vi "Main.vi"(8 "error in":errorcluster, 11 "gRPC Client Tester in":refnum<class "gRPC Client Tester.lvclass">) -> (0 "error out":errorcluster, 3 "gRPC Client Tester out":refnum<class "gRPC Client Tester.lvclass">)   [LabVIEW 2019, in "gRPC Client Tester.lvclass"]
doc: "The <b>Queued Message Handler</b> of the Worker that owns this VI."
uses:
  gRPC Client Tester.lvclass
  C:/Program Files (x86)/National Instruments/LabVIEW 2019/vi.lib/addons/_Workers/Library/Classes/Worker/Worker.lvclass
  Generated_client/RPC Messages/w4lvgrpc_Msg_ToServer_4.ctl
  Generated_client/RPC Messages/w4lvgrpc_Msg_ToServer_1.ctl
  Generated_client/RPC Messages/w4lvgrpc_Msg_ToServer_2.ctl
  Generated_client/RPC Messages/w4lvgrpc_Msg_ToServer_3.ctl
  Generated_client/RPC Messages/w4lvgrpc_Msg_ToServer_5.ctl
  Generated_client/RPC Messages/w4lvgrpc_Msg_ToClient_1.ctl
  Generated_client/RPC Messages/w4lvgrpc_Msg_ToClient_2.ctl
  Generated_client/RPC Messages/w4lvgrpc_Msg_ToClient_3.ctl
  Generated_client/RPC Messages/w4lvgrpc_Msg_ToClient_4.ctl
  Generated_client/RPC Messages/w4lvgrpc_Msg_ToClient_5.ctl
  gRPC Client Tester.lvclass/gRPC Client Tester.ctl
  gRPC Client/gRPC Client/rqp_Msg_ToServer_1.ctl
  gRPC Client/gRPC Client/rqp_Msg_ToServer_2.ctl
  gRPC Client/gRPC Client/rqp_Msg_ToServer_3.ctl
  gRPC Client/gRPC Client/rqp_Msg_ToServer_4.ctl
  gRPC Client/gRPC Client/rqp_Msg_ToServer_5.ctl
  Initialization Data.ctl
  Response Cases.ctl
  rql_Create gRPC Client.ctl
  gRPC Client/gRPC Client/rwr_Create gRPC Client.ctl
  rql_Destroy gRPC Client.ctl
  <vilib>/addons/_Workers/Library/Classes/Message Queue/Message Queue.lvclass
  gRPC Client/gRPC Client/gRPC Client.lvclass
  Generated_client/Generated_client.lvlib
panel:
  out "Msg_ToClient_5":T1
  out "Msg_ToClient_4":T2
  out "Msg_ToClient_3":T3
  out "Msg_ToClient_2":T4
  out "Msg_ToClient_1":T5
  in  "Msg_ToServer_5":T6
  in  "Msg_ToServer_3":T7
  in  "Msg_ToServer_2":T8
  in  "Msg_ToServer_1":T9
  in  "Msg_ToServer_4":T10
  out "gRPC ID":u64
  out "Client Connected":bool
  in  "Server Address":string="localhost:50070"
  in  "Destroy gRPC Client":bool
  in  "Create gRPC Client":bool
  # "gRPC Client Worker - Public Requests"
  # "Messages Client -> Server"
  # "gRPC Client Worker Template Tester"
  # "Instructions:\n\nSee project file called Readme.md"
  # "gRPC Client Worker - Public Responses"
  # "Messages Server -> Client"
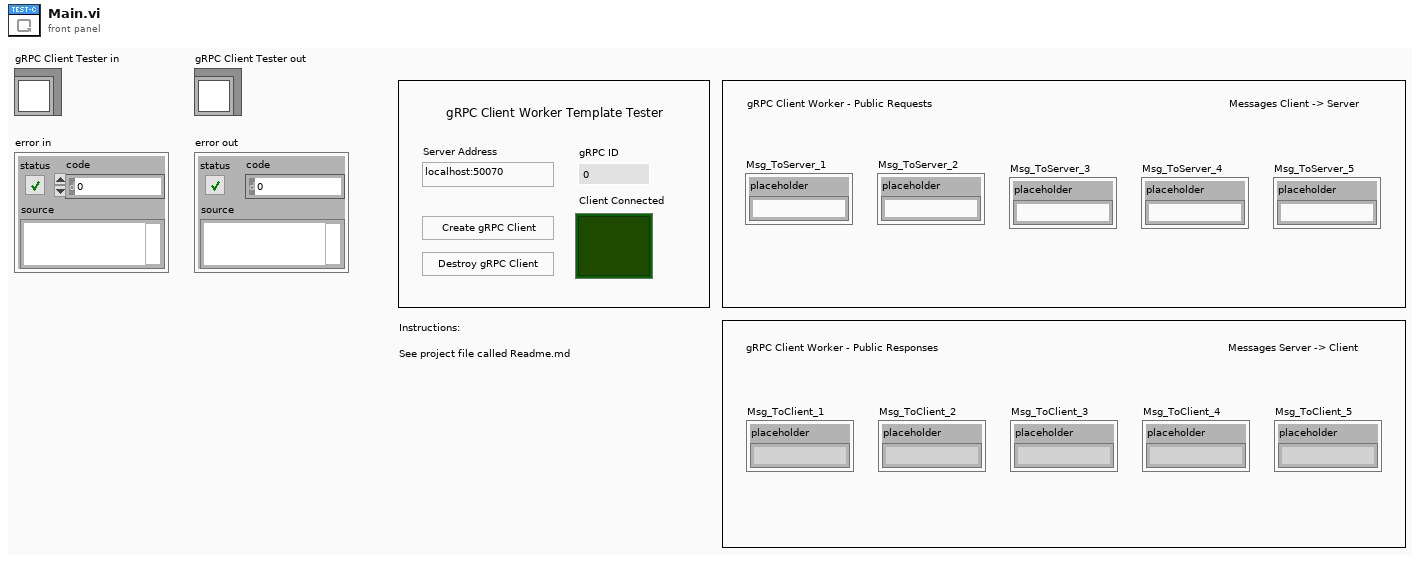
[diagram p1: front panel]
types:
  T1 = typedef "Generated_client.lvlib/w4lvgrpc_Msg_ToClient_5.ctl" = cluster{"placeholder":string}
  T2 = typedef "Generated_client.lvlib/w4lvgrpc_Msg_ToClient_4.ctl" = cluster{"placeholder":string}
  T3 = typedef "Generated_client.lvlib/w4lvgrpc_Msg_ToClient_3.ctl" = cluster{"placeholder":string}
  T4 = typedef "Generated_client.lvlib/w4lvgrpc_Msg_ToClient_2.ctl" = cluster{"placeholder":string}
  T5 = typedef "Generated_client.lvlib/w4lvgrpc_Msg_ToClient_1.ctl" = cluster{"placeholder":string}
  T6 = typedef "Generated_client.lvlib/w4lvgrpc_Msg_ToServer_5.ctl" = cluster{"placeholder":string}
  T7 = typedef "Generated_client.lvlib/w4lvgrpc_Msg_ToServer_3.ctl" = cluster{"placeholder":string}
  T8 = typedef "Generated_client.lvlib/w4lvgrpc_Msg_ToServer_2.ctl" = cluster{"placeholder":string}
  T9 = typedef "Generated_client.lvlib/w4lvgrpc_Msg_ToServer_1.ctl" = cluster{"placeholder":string}
  T10 = typedef "Generated_client.lvlib/w4lvgrpc_Msg_ToServer_4.ctl" = cluster{"placeholder":string}
  T11 = typedef "gRPC Client Tester.lvclass/Initialization Data.ctl" = cluster{"Response Cases":T12}
  T12 = typedef "gRPC Client Tester.lvclass/Response Cases.ctl" = cluster{"Placeholder - Can be deleted":string}
  T13 = typedef "gRPC Client Tester.lvclass/rql_Create gRPC Client.ctl" = cluster{"String":string}
  T14 = typedef "gRPC Client (template.proto).lvlib/gRPC Client.lvclass/rwr_Create gRPC Client.ctl" = cluster{"Server Address":string, "Certificate Path":string}
  T15 = typedef "gRPC Client Tester.lvclass/rql_Destroy gRPC Client.ctl" = cluster{"String":string}
  T16 = typedef "gRPC Client (template.proto).lvlib/gRPC Client.lvclass/rqp_Msg_ToServer_1.ctl" = cluster{"w4lvgrpc_Msg_ToServer_1":T9}
  T17 = typedef "gRPC Client (template.proto).lvlib/gRPC Client.lvclass/rqp_Msg_ToServer_2.ctl" = cluster{"w4lvgrpc_Msg_ToServer_2":T8}
  T18 = typedef "gRPC Client (template.proto).lvlib/gRPC Client.lvclass/rqp_Msg_ToServer_3.ctl" = cluster{"w4lvgrpc_Msg_ToServer_3":T7}
  T19 = typedef "gRPC Client (template.proto).lvlib/gRPC Client.lvclass/rqp_Msg_ToServer_4.ctl" = cluster{"w4lvgrpc_Msg_ToServer_4":T10}
  T20 = typedef "gRPC Client (template.proto).lvlib/gRPC Client.lvclass/rqp_Msg_ToServer_5.ctl" = cluster{"w4lvgrpc_Msg_ToServer_5":T6}
  T21 = typedef "gRPC Client (template.proto).lvlib/gRPC Client.lvclass/rsp_Connection Notify.ctl" = cluster{"gRPC ID":T22, "Connected?":bool}
  T22 = typedef "grpc-lvsupport-release.lvlib/grpcId.ctl" = u64
  T23 = typedef "gRPC Client (template.proto).lvlib/gRPC Client.lvclass/rsp_Client Error.ctl" = errorcluster
  T24 = typedef "gRPC Client (template.proto).lvlib/gRPC Client.lvclass/rsp_Msg_ToClient_1.ctl" = cluster{"w4lvgrpc_Msg_ToClient_1":T5}
  T25 = typedef "gRPC Client (template.proto).lvlib/gRPC Client.lvclass/rsp_Msg_ToClient_2.ctl" = cluster{"w4lvgrpc_Msg_ToClient_2":T4}
  T26 = typedef "gRPC Client (template.proto).lvlib/gRPC Client.lvclass/rsp_Msg_ToClient_3.ctl" = cluster{"w4lvgrpc_Msg_ToClient_3":T3}
  T27 = typedef "gRPC Client (template.proto).lvlib/gRPC Client.lvclass/rsp_Msg_ToClient_4.ctl" = cluster{"w4lvgrpc_Msg_ToClient_4":T2}
  T28 = typedef "gRPC Client (template.proto).lvlib/gRPC Client.lvclass/rsp_Msg_ToClient_5.ctl" = cluster{"w4lvgrpc_Msg_ToClient_5":T1}
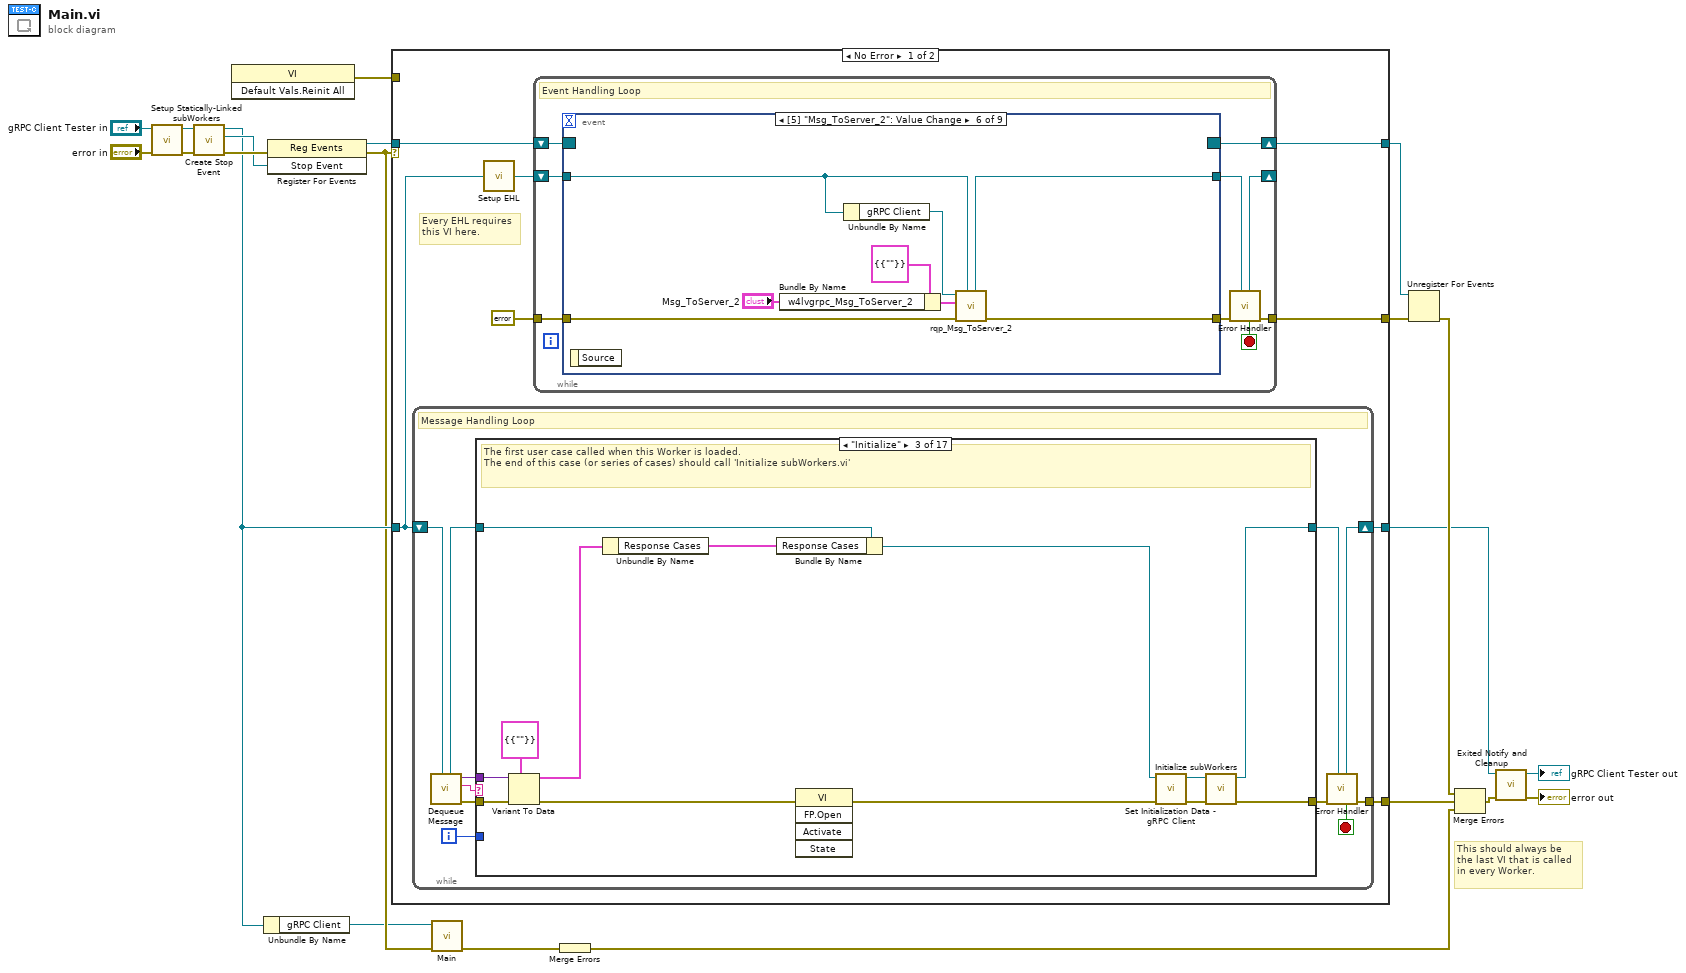
[diagram p0: block diagram]
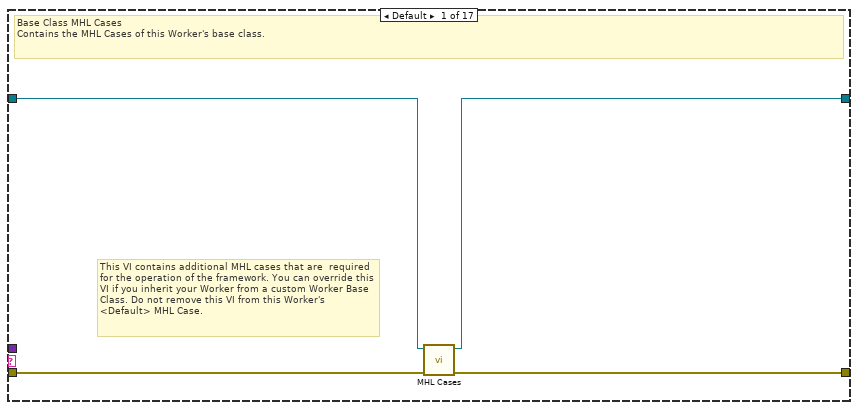
[diagram p2: hidden frame]
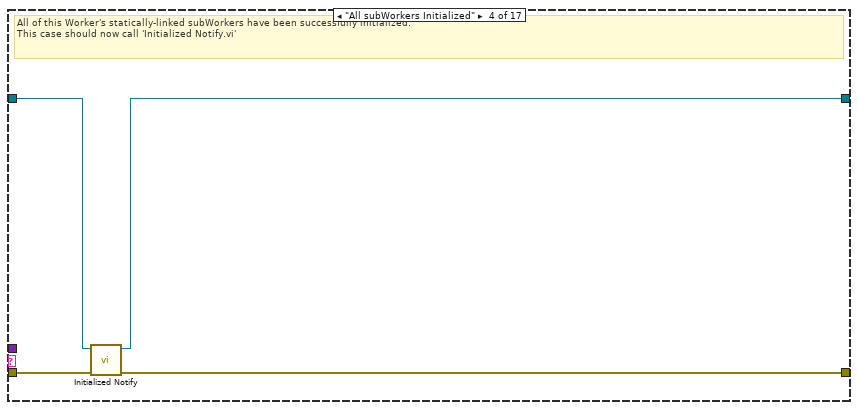
[diagram p4: hidden frame]
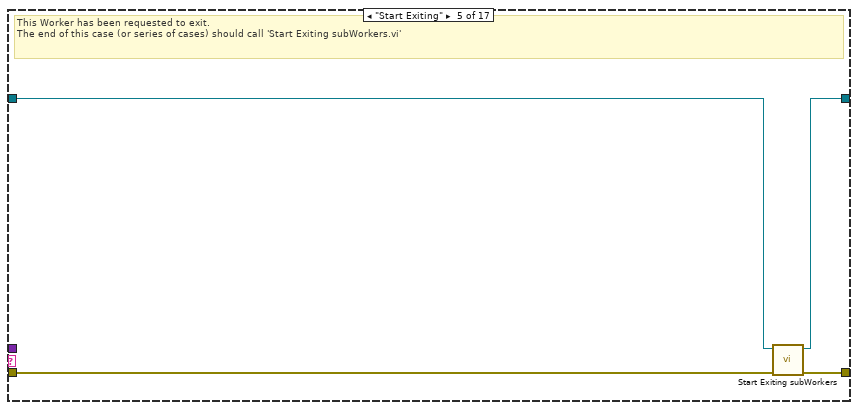
[diagram p5: hidden frame]
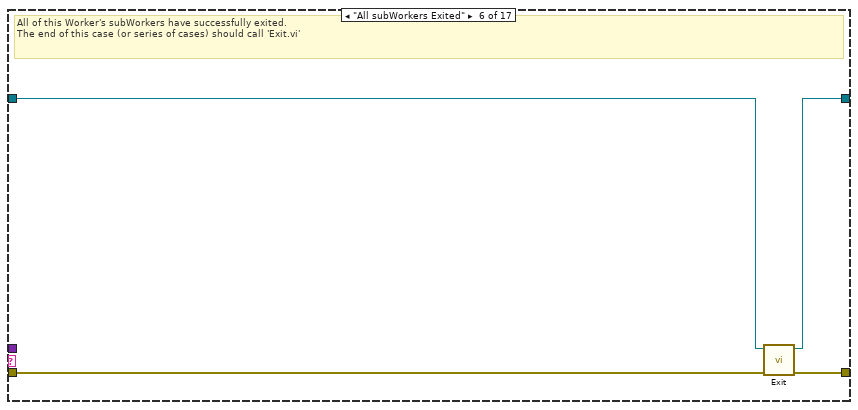
[diagram p6: hidden frame]
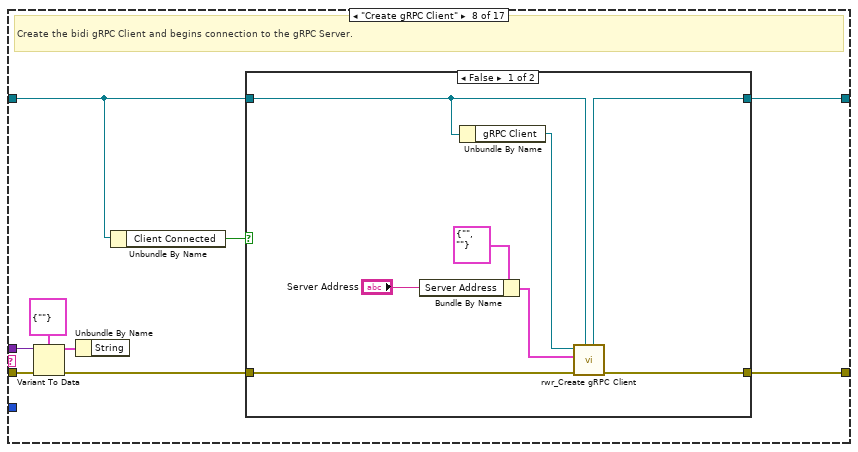
[diagram p8: hidden frame]
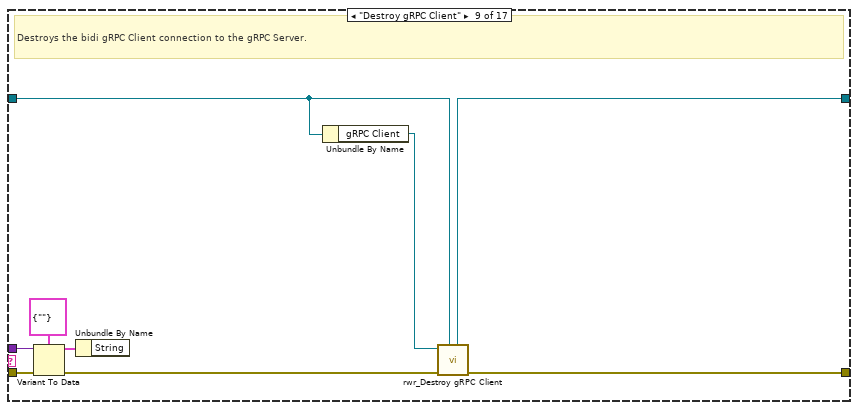
[diagram p10: hidden frame]
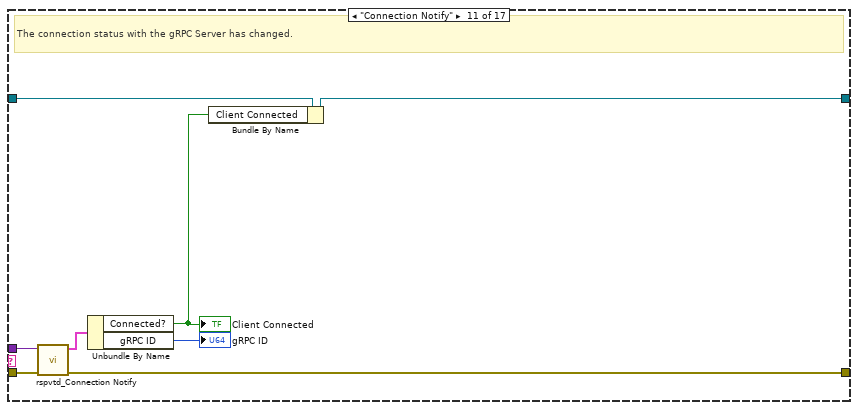
[diagram p12: hidden frame]
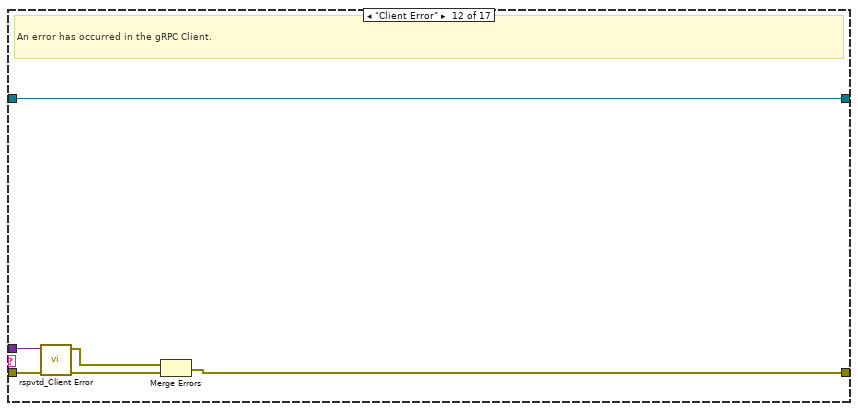
[diagram p13: hidden frame]
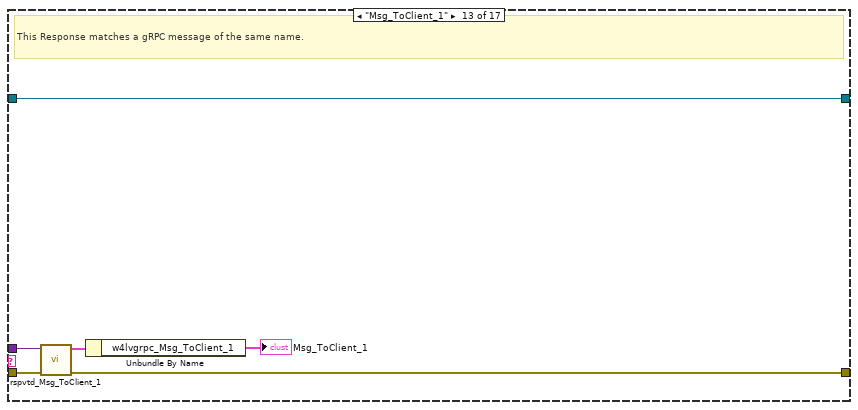
[diagram p14: hidden frame]
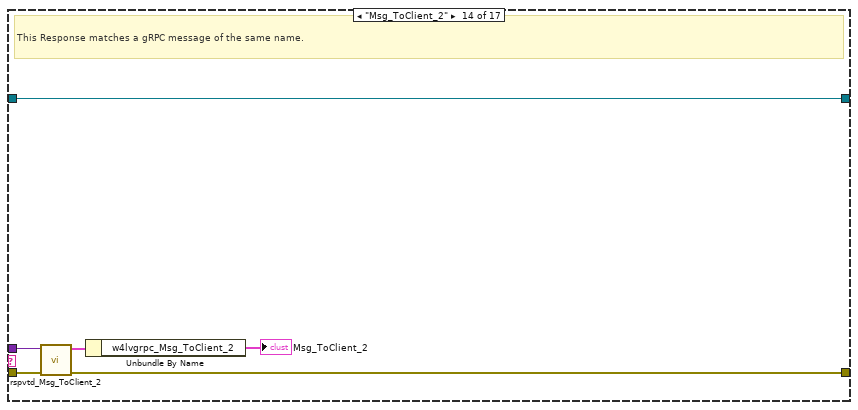
[diagram p15: hidden frame]
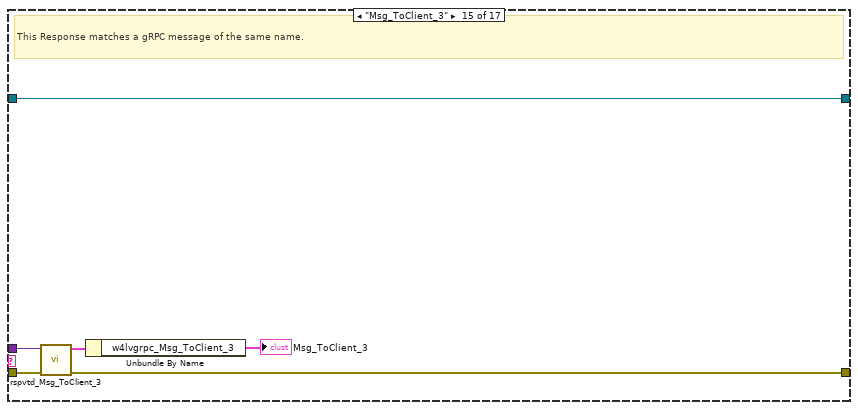
[diagram p16: hidden frame]
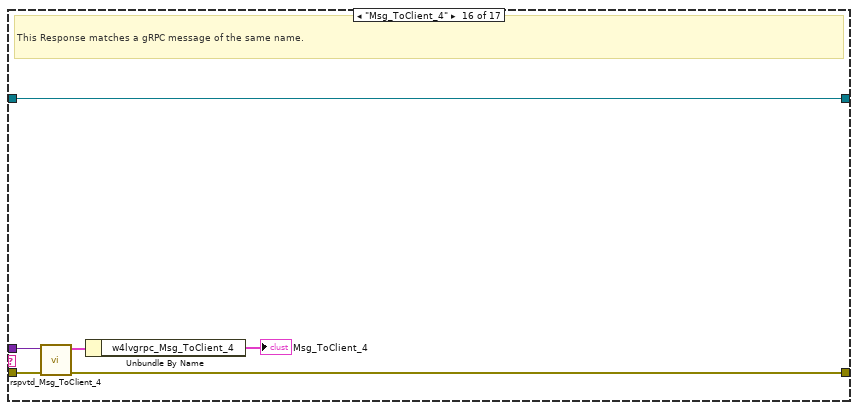
[diagram p17: hidden frame]
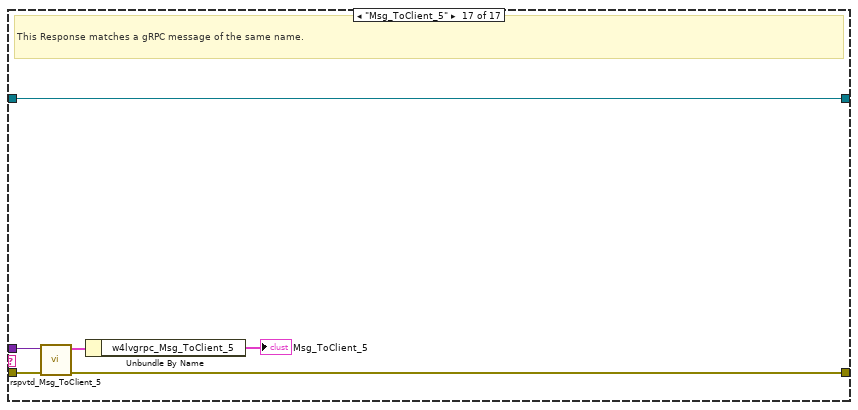
[diagram p18: hidden frame]
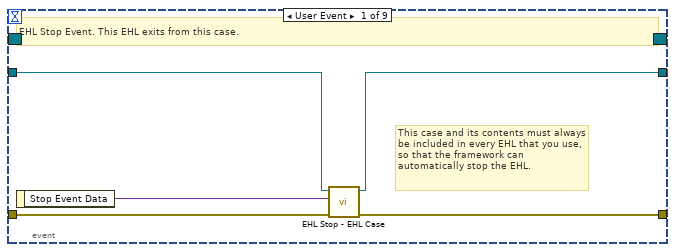
[diagram p19: hidden frame]
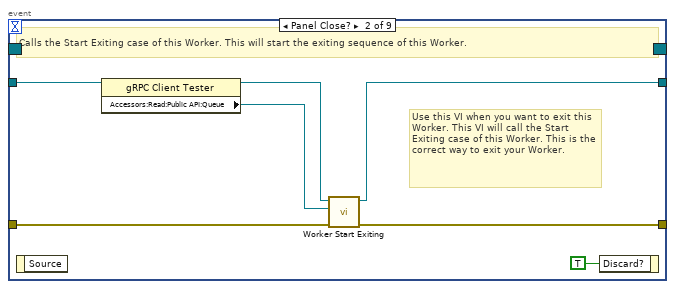
[diagram p20: hidden frame]
diagram:
  # "This should always be the last VI that is called in every Worker."
  n1 = call "Setup Statically-Linked subWorkers.vi"("error in"="error in", "gRPC Client Tester in"="gRPC Client Tester in") -> ("error out"=w6:errorcluster, "gRPC Client Tester out"=w4:refnum<class "gRPC Client Tester.lvclass">)  [unwired: 8 in]
  n2 = call-dynamic "Create Stop Event.vi"("error in"=w6, "Worker"=w4) -> ("error out"=w16:errorcluster, "Stop Event"=w13:refnum<user-event>, "Worker out"=w10:refnum<class "gRPC Client Tester.lvclass">)  [unwired: 7 in]
  n3 = invoke class="VI" method="Default Vals.Reinit All"() -> (error out=w8:errorcluster)  [unwired: 3 in, 2 out]
  n4 = Unbundle By Name(w10) -> ("gRPC Client"=w1:refnum<class "gRPC Client.lvclass">)
  n5 = register-events(error in=w16, w13) -> (reference out=w15:refnum<event-registration>, error out=w9:errorcluster)  [unwired: 1 in]
  n6 = case shown="No Error" w9 {
    tunnel: w10 -> [w24 w218]
    tunnel: [w22 w219] -> w14
    tunnel: w15 -> [w29 w220]
    tunnel: [w26 w221] -> w20
    tunnel: [w28 w220] -> w19
    tunnel: [w23 w217] -> w17
    selector: w9 -> [_ w221]
    tunnel: w8 -> [_ _]
    frame No Error {
      # "Every EHL requires\nthis VI here."
      n7 = while {
        shift-right: [w38] -> w23
        shift-left: w24 -> [w40]
        tunnel: [w39] -> w22
        i -> [w31]
        stop <- w32 stop-if-true
        # "Message Handling Loop"
        n8 = call-dynamic "Dequeue Message.vi"("Worker"=w40) -> ("error out"=w37:errorcluster, "Case out"=w33:string, "Data out"=w30:variant, "Worker out"=w35:refnum<class "gRPC Client Tester.lvclass">)  [unwired: 6 in, 1 out]
        n9 = case "Worker MHL Case Structure (DO NOT CHANGE LABEL NAME)" shown="\"Initialize\"" w33 {
          tunnel: w37 -> [w44 w45 w57 w62 w64 w71 w73 w82 w101 w103 w111 w117 w123 w129 w135 w141 w147]
          tunnel: [w43 w45 w59 w60 w67 w70 w73 w77 w96 w103 w104 w113 w121 w127 w133 w139 w145] -> w36
          tunnel: w35 -> [w42 w46 w56 w63 w65 w69 w72 w75 w94 w102 w110 w116 w122 w128 w134 w140 w146]
          tunnel: [w41 w46 w58 w61 w66 w68 w72 w76 w95 w102 w105 w116 w122 w128 w134 w140 w146] -> w34
          tunnel: w31 -> [_ _ _ _ _ _ _ _ _ _ _ _ _ _ _ _ _]
          tunnel: w30 -> [_ _ w55 _ _ _ _ w79 w98 _ w109 w114 w120 w126 w132 w138 w144]
          frame Default {
            # "This VI contains additional MHL cases that are  required for the operation of the framework. You can override this VI if you inherit your Worker from a custom Worker Base Class. Do not remove this VI from this Worker's <Default> MHL Case."
            # "Base Class MHL Cases\nContains the MHL Cases of this Worker's base class."
            n10 = call-dynamic "MHL Cases.vi"("error in"=w44, "Worker in"=w42) -> ("error out"=w43:errorcluster, "Worker out"=w41:refnum<class "gRPC Client Tester.lvclass">)  [unwired: 8 in]
          }
          frame "------------ FRAMEWORK CASES -----------" {
            # "Start of Workers Framework Cases"
          }
          frame "Initialize" {
            # "The first user case called when this Worker is loaded.\nThe end of this case (or series of cases) should call 'Initialize subWorkers.vi'"
            n11 = Variant To Data(error in=w57, type=T11 {"Response Cases"={"Placeholder - Can be deleted"=""}} ("Initialization Data"), Variant=w55) -> (data=w54:T11, error out=w48:errorcluster)
            n12 = Unbundle By Name(w54) -> ("Response Cases"=w53:T12)
            n13 = Bundle By Name(cluster=w56, "Response Cases"=w53) -> (w49:refnum<class "gRPC Client Tester.lvclass">)
            n14 = invoke class="VI" method="FP.Open"(error in=w48) -> (error out=w47:errorcluster)  [unwired: 4 in, 4 out]
            n15 = call "Set Initialization Data - gRPC Client.vi"("error in"=w47, "gRPC Client Tester in"=w49) -> ("error out"=w51:errorcluster, "gRPC Client Tester out"=w50:refnum<class "gRPC Client Tester.lvclass">)  [unwired: 8 in]
            n16 = call-dynamic "Initialize subWorkers.vi"("error in"=w51, "Worker"=w50) -> ("error out"=w59:errorcluster, "dup Worker out"=w58:refnum<class "gRPC Client Tester.lvclass">)  [unwired: 8 in]
          }
          frame "All subWorkers Initialized" {
            # "All of this Worker's statically-linked subWorkers have been successfully initialized.\nThis case should now call 'Initialized Notify.vi'"
            n17 = call-dynamic "Initialized Notify.vi"("error in"=w62, "Worker"=w63) -> ("error out"=w60:errorcluster, "dup Worker out"=w61:refnum<class "gRPC Client Tester.lvclass">)  [unwired: 8 in]
          }
          frame "Start Exiting" {
            # "This Worker has been requested to exit. \nThe end of this case (or series of cases) should call 'Start Exiting subWorkers.vi'"
            n18 = call-dynamic "Start Exiting subWorkers.vi"("error_in"=w64, "Worker"=w65) -> ("error out"=w67:errorcluster, "dup Worker out"=w66:refnum<class "gRPC Client Tester.lvclass">)  [unwired: 8 in]
          }
          frame "All subWorkers Exited" {
            # "All of this Worker's subWorkers have successfully exited. \nThe end of this case (or series of cases) should call 'Exit.vi'"
            n19 = call-dynamic "Exit.vi"("error_in"=w71, "Worker"=w69) -> ("error out"=w70:errorcluster, "dup Worker out"=w68:refnum<class "gRPC Client Tester.lvclass">)  [unwired: 8 in]
          }
          frame "------------- LOCAL API CASES -------------" {
            # "Start of Workers Local API Cases"
          }
          frame "Create gRPC Client" {
            # "Create the bidi gRPC Client and begins connection to the gRPC Server."
            n20 = Variant To Data(error in=w82, type=T13 {"String"=""} ("Data"), Variant=w79) -> (data=w78:T13, error out=w81:errorcluster)
            n21 = Unbundle By Name(w78) -> ()  [unwired: 1 out]
            n22 = Unbundle By Name(w75) -> ("Client Connected"=w74:bool)
            n23 = case shown="False" w74 {
              tunnel: w81 -> [w90 w91]
              tunnel: [w89 w91] -> w77
              tunnel: [w88 w92] -> w76
              tunnel: w75 -> [w87 w92]
              frame False {
                n24 = Bundle By Name(cluster=T14 {"Server Address"="", "Certificate Path"=""} ("Data in"), "Server Address"="Server Address") -> (w84:T14)
                n25 = Unbundle By Name(w87) -> ("gRPC Client"=w86:refnum<class "gRPC Client.lvclass">)
                n26 = call "rwr_Create gRPC Client.vi"("Caller in"=w87, "error in"=w90, "Data in"=w84, "gRPC Client in"=w86) -> ("error out"=w89:errorcluster, "dup Caller out"=w88:refnum<class "gRPC Client Tester.lvclass">)  [unwired: 4 in, 2 out]
              }
              frame True {
                # "gRPC Client is already connected to gRPC Server. Nothing to do."
              }
            }
          }
          frame "Destroy gRPC Client" {
            # "Destroys the bidi gRPC Client connection to the gRPC Server."
            n27 = Variant To Data(error in=w101, type=T15 {"String"=""} ("Data"), Variant=w98) -> (data=w97:T15, error out=w100:errorcluster)
            n28 = Unbundle By Name(w97) -> ()  [unwired: 1 out]
            n29 = Unbundle By Name(w94) -> ("gRPC Client"=w93:refnum<class "gRPC Client.lvclass">)
            n30 = call "rwr_Destroy gRPC Client.vi"("Caller in"=w94, "error in"=w100, "gRPC Client in"=w93) -> ("error out"=w96:errorcluster, "dup Caller out"=w95:refnum<class "gRPC Client Tester.lvclass">)  [unwired: 5 in, 2 out]
          }
          frame "------------- RESPONSE CASES --------------" {
            # "Start of Workers Response Cases"
          }
          frame "Connection Notify" {
            # "The connection status with the gRPC Server has changed."
            n31 = call "rspvtd_Connection Notify.vi"("error in"=w111, "Data in"=w109) -> ("error out"=w104:errorcluster, "Data out"=w108:T21)  [unwired: 8 in]
            n32 = Unbundle By Name(w108) -> ("Connected?"=w107:bool, "gRPC ID"=→"gRPC ID":T22)
            "Client Connected" <- w107
            n33 = Bundle By Name(cluster=w110, "Client Connected"=w107) -> (w105:refnum<class "gRPC Client Tester.lvclass">)
          }
          frame "Client Error" {
            # "An error has occurred in the gRPC Client."
            n34 = call "rspvtd_Client Error.vi"("error in"=w117, "Data in"=w114) -> ("error out"=w115:errorcluster, "Data out"=w112:T23)  [unwired: 8 in]
            n35 = Merge Errors(w112, w115) -> (w113:errorcluster)
          }
          frame "Msg_ToClient_1" {
            # "This Response matches a gRPC message of the same name."
            n36 = call "rspvtd_Msg_ToClient_1.vi"("error in"=w123, "Data in"=w120) -> ("error out"=w121:errorcluster, "Data out"=w119:T24)  [unwired: 8 in]
            n37 = Unbundle By Name(w119) -> ("w4lvgrpc_Msg_ToClient_1"=→"Msg_ToClient_1":T5)
          }
          frame "Msg_ToClient_2" {
            # "This Response matches a gRPC message of the same name."
            n38 = call "rspvtd_Msg_ToClient_2.vi"("error in"=w129, "Data in"=w126) -> ("error out"=w127:errorcluster, "Data out"=w125:T25)  [unwired: 8 in]
            n39 = Unbundle By Name(w125) -> ("w4lvgrpc_Msg_ToClient_2"=→"Msg_ToClient_2":T4)
          }
          frame "Msg_ToClient_3" {
            # "This Response matches a gRPC message of the same name."
            n40 = call "rspvtd_Msg_ToClient_3.vi"("error in"=w135, "Data in"=w132) -> ("error out"=w133:errorcluster, "Data out"=w131:T26)  [unwired: 8 in]
            n41 = Unbundle By Name(w131) -> ("w4lvgrpc_Msg_ToClient_3"=→"Msg_ToClient_3":T3)
          }
          frame "Msg_ToClient_4" {
            # "This Response matches a gRPC message of the same name."
            n42 = call "rspvtd_Msg_ToClient_4.vi"("error in"=w141, "Data in"=w138) -> ("error out"=w139:errorcluster, "Data out"=w137:T27)  [unwired: 8 in]
            n43 = Unbundle By Name(w137) -> ("w4lvgrpc_Msg_ToClient_4"=→"Msg_ToClient_4":T2)
          }
          frame "Msg_ToClient_5" {
            # "This Response matches a gRPC message of the same name."
            n44 = call "rspvtd_Msg_ToClient_5.vi"("error in"=w147, "Data in"=w144) -> ("error out"=w145:errorcluster, "Data out"=w143:T28)  [unwired: 8 in]
            n45 = Unbundle By Name(w143) -> ("w4lvgrpc_Msg_ToClient_5"=→"Msg_ToClient_5":T1)
          }
        }
        n46 = call-dynamic "Error Handler.vi"("Worker"=w34, "error_in"=w36) -> ("error out"=w39:errorcluster, "Stop Loop"=w32:bool, "Worker out"=w38:refnum<class "gRPC Client Tester.lvclass">)  [unwired: 7 in]
      }
      n47 = call-dynamic "Setup EHL.vi"("Worker"=w24) -> ("Worker out"=w25:refnum<class "gRPC Client Tester.lvclass">)  [unwired: 14 in]
      n48 = while "Event Handling Loop" {
        shift-right: [w156] -> w28
        shift-left: w29 -> [w155]
        tunnel: [w151] -> w26
        tunnel: errorcluster {"status"=FALSE, "code"=0, "source"=""} ("error constant") -> [w153]
        shift-right: [w149] -> _
        shift-left: w25 -> [w154]
        stop <- w148 stop-if-true
        # "Event Handling Loop"
        n49 = event shown="[5] \"Msg_ToServer_2\": Value Change" {
          selector: w155 -> [_ _ _ _ _ _ _ _ _]
          dyn-events: [_ _ _ _ _ _ _ _ _] -> w156
          timeout: _ -> [_ _ _ _ _ _ _ _ _]
          tunnel: [w160 w167 w171 w175 w183 w191 w199 w207 w215] -> w152
          tunnel: w153 -> [w161 w166 w172 w176 w184 w192 w200 w208 w216]
          tunnel: w154 -> [w159 w165 w170 w174 w179 w187 w195 w203 w211]
          tunnel: [w158 w164 w169 w173 w182 w190 w198 w206 w214] -> w150
          event User Event {
            # "This case and its contents must always be included in every EHL that you use, so that the framework can automatically stop the EHL."
            # "EHL Stop Event. This EHL exits from this case."
            n50 = event-data() -> ("Stop Event Data"=w157:variant)  [unwired: 1 in]
            n51 = call-dynamic "EHL Stop - EHL Case.vi"("error in"=w161, "Stop Event Data"=w157, "Worker"=w159) -> ("error out"=w160:errorcluster, "Worker out"=w158:refnum<class "gRPC Client Tester.lvclass">)  [unwired: 7 in]
          }
          event Panel Close? {
            # "Use this VI when you want to exit this Worker. This VI will call the Start Exiting case of this Worker. This is the correct way to exit your Worker."
            # "Calls the Start Exiting case of this Worker. This will start the exiting sequence of this Worker."
            n52 = event-data() -> ()  [unwired: 1 in, 1 out]
            n53 = property class="gRPC Client Tester"(reference=w165) -> (reference out=w163:refnum<class "gRPC Client Tester.lvclass">, "Accessors:Read:Public API:Queue"=w162:refnum<class "Message Queue.lvclass">)  [unwired: 1 in, 1 out]
            n54 = call-dynamic "Worker Start Exiting.vi"("error_in"=w166, "Message Queue"=w162, "Worker"=w163) -> ("error out"=w167:errorcluster, "dup Worker out"=w164:refnum<class "gRPC Client Tester.lvclass">)  [unwired: 7 in]
            n55 = event-data ("Event Filter Node")("Discard?"=TRUE) -> ()  [unwired: 1 in, 1 out]
          }
          event "Create gRPC Client": Value Change {
            n56 = event-data() -> ()  [unwired: 1 in, 1 out]
            n57 = call "rql_Create gRPC Client.vi"("error in"=w172, "gRPC Client Tester in"=w170) -> ("error out"=w171:errorcluster, "dup gRPC Client Tester out"=w169:refnum<class "gRPC Client Tester.lvclass">)  [unwired: 8 in]
          }
          event "Destroy gRPC Client": Value Change {
            n58 = event-data() -> ()  [unwired: 1 in, 1 out]
            n59 = call "rql_Destroy gRPC Client.vi"("error in"=w176, "gRPC Client Tester in"=w174) -> ("error out"=w175:errorcluster, "dup gRPC Client Tester out"=w173:refnum<class "gRPC Client Tester.lvclass">)  [unwired: 8 in]
          }
          event Value Change {
            n60 = event-data() -> ()  [unwired: 1 in, 1 out]
            n61 = Bundle By Name(cluster=T16 {"w4lvgrpc_Msg_ToServer_1"={"placeholder"=""}} ("Data in"), "w4lvgrpc_Msg_ToServer_1"="Msg_ToServer_1") -> (w180:T16)
            n62 = Unbundle By Name(w179) -> ("gRPC Client"=w178:refnum<class "gRPC Client.lvclass">)
            n63 = call "rqp_Msg_ToServer_1.vi"("Caller in"=w179, "error in"=w184, "Data in"=w180, "gRPC Client in"=w178) -> ("error out"=w183:errorcluster, "dup Caller out"=w182:refnum<class "gRPC Client Tester.lvclass">)  [unwired: 5 in, 1 out]
          }
          event Value Change {
            n64 = event-data() -> ()  [unwired: 1 in, 1 out]
            n65 = Bundle By Name(cluster=T17 {"w4lvgrpc_Msg_ToServer_2"={"placeholder"=""}} ("Data in"), "w4lvgrpc_Msg_ToServer_2"="Msg_ToServer_2") -> (w188:T17)
            n66 = Unbundle By Name(w187) -> ("gRPC Client"=w186:refnum<class "gRPC Client.lvclass">)
            n67 = call "rqp_Msg_ToServer_2.vi"("Caller in"=w187, "error in"=w192, "Data in"=w188, "gRPC Client in"=w186) -> ("error out"=w191:errorcluster, "dup Caller out"=w190:refnum<class "gRPC Client Tester.lvclass">)  [unwired: 5 in, 1 out]
          }
          event Value Change {
            n68 = event-data() -> ()  [unwired: 1 in, 1 out]
            n69 = Bundle By Name(cluster=T18 {"w4lvgrpc_Msg_ToServer_3"={"placeholder"=""}} ("Data in"), "w4lvgrpc_Msg_ToServer_3"="Msg_ToServer_3") -> (w196:T18)
            n70 = Unbundle By Name(w195) -> ("gRPC Client"=w194:refnum<class "gRPC Client.lvclass">)
            n71 = call "rqp_Msg_ToServer_3.vi"("Caller in"=w195, "error in"=w200, "Data in"=w196, "gRPC Client in"=w194) -> ("error out"=w199:errorcluster, "dup Caller out"=w198:refnum<class "gRPC Client Tester.lvclass">)  [unwired: 5 in, 1 out]
          }
          event Value Change {
            n72 = event-data() -> ()  [unwired: 1 in, 1 out]
            n73 = Bundle By Name(cluster=T19 {"w4lvgrpc_Msg_ToServer_4"={"placeholder"=""}} ("Data in"), "w4lvgrpc_Msg_ToServer_4"="Msg_ToServer_4") -> (w204:T19)
            n74 = Unbundle By Name(w203) -> ("gRPC Client"=w202:refnum<class "gRPC Client.lvclass">)
            n75 = call "rqp_Msg_ToServer_4.vi"("Caller in"=w203, "error in"=w208, "Data in"=w204, "gRPC Client in"=w202) -> ("error out"=w207:errorcluster, "dup Caller out"=w206:refnum<class "gRPC Client Tester.lvclass">)  [unwired: 5 in, 1 out]
          }
          event Value Change {
            n76 = event-data() -> ()  [unwired: 1 in, 1 out]
            n77 = Bundle By Name(cluster=T20 {"w4lvgrpc_Msg_ToServer_5"={"placeholder"=""}} ("Data in"), "w4lvgrpc_Msg_ToServer_5"="Msg_ToServer_5") -> (w212:T20)
            n78 = Unbundle By Name(w211) -> ("gRPC Client"=w210:refnum<class "gRPC Client.lvclass">)
            n79 = call "rqp_Msg_ToServer_5.vi"("Caller in"=w211, "error in"=w216, "Data in"=w212, "gRPC Client in"=w210) -> ("error out"=w215:errorcluster, "dup Caller out"=w214:refnum<class "gRPC Client Tester.lvclass">)  [unwired: 5 in, 1 out]
          }
        }
        n80 = call-dynamic "Error Handler.vi"("Worker"=w150, "error_in"=w152) -> ("error out"=w151:errorcluster, "Stop Loop"=w148:bool, "Worker out"=w149:refnum<class "gRPC Client Tester.lvclass">)  [unwired: 7 in]
      }
    }
    frame Error {
      n81 = call-dynamic "Error Handler.vi"("Worker"=w218, "error_in"=w221) -> ("error out"=w219:errorcluster, "Worker out"=w217:refnum<class "gRPC Client Tester.lvclass">)  [unwired: 7 in, 1 out]
    }
  }
  n82 = call-dynamic "Main.vi"("error in"=w9, "gRPC Client in"=w1) -> ("error out"=w3:errorcluster)  [unwired: 8 in, 1 out]
  n83 = Merge Errors(w3) -> (w2:errorcluster)
  n84 = Unregister For Events(event registration refnum=w19, error in=w20) -> (error out=w21:errorcluster)
  n85 = Merge Errors(w21, w14, w2) -> (w18:errorcluster)
  n86 = call-dynamic "Exited Notify and Cleanup.vi"("error_in"=w18, "Worker"=w17) -> ("error out"=→"error out":errorcluster, "dup Worker out"=→"gRPC Client Tester out":refnum<class "gRPC Client Tester.lvclass">)  [unwired: 8 in]
